vi "Disabled.vi"(7 "Robot Mode":T2, 10 "Match Info":T1={"Autonomous Elapsed Seconds"=0.0, "TeleOp Elapsed Seconds"=0.0, "Disabled Elapsed Seconds"=0.0, "Visited Autonomous"=FALSE, "Visited TeleOp"=FALSE, "Visited Disabled"=FALSE, "Autonomous Settings"={"Autonomous Style"=enum."Independent", "VI Refnum"=refnum}}, 11 "Call Context":T3) -> ()   [LabVIEW 2014]
doc: "This VI is called each time a disabled packet is received from the DS. It is often used to prepare for the next robot mode, to calibrate sensors, etc."
uses:
  <vilib>/Rock Robotics/WPI/DriverStation/WPI_DriverStationDerivedRobotMode.ctl
  <vilib>/Rock Robotics/WPI/DriverStation/WPI_DriverStationRobotMode2.ctl
  <vilib>/Rock Robotics/WPI/DriverStation/WPI_DriverStationMatch Info.ctl
  Raw Sequence Cluster.ctl
  LED Message.ctl
  LED_Patterns.ctl
  LED_Colors.ctl
  <vilib>/NI/AMC/Create Single Message.vi
  <vilib>/NI/AMC/Update Message Routing Info.vi
  <vilib>/NI/AMC/Send Message.vi
  <vilib>/Rock Robotics/WPI/Joystick/WPI_JoystickGetSetRefNum.vi
  <vilib>/NI/AMC/AMC.lvlib
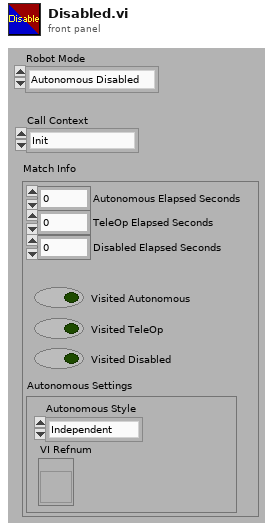
[diagram p1: front panel]
types:
  T1 = typedef "WPI_DriverStationMatch Info.ctl" = cluster{"Autonomous Elapsed Seconds":dbl, "TeleOp Elapsed Seconds":dbl, "Disabled Elapsed Seconds":dbl, "Visited Autonomous":bool, "Visited TeleOp":bool, "Visited Disabled":bool, "Autonomous Settings":cluster{"Autonomous Style":enum16{"Iterative", "Independent"}, "VI Refnum":refnum<vi>}}
  T2 = typedef "WPI_DriverStationRobotMode2.ctl" = enum16{"Autonomous Disabled", "Autonomous Enabled", "Teleop Disabled", "Teleop Enabled", "Disconnected", "Finish", "Test Disabled", "Test Enabled", "Emergency Stopped"}
  T3 = typedef "WPI_DriverStationDerivedRobotMode.ctl" = enum16{"Init", "Execute", "Stop"}
  T4 = typedef "Raw Sequence Cluster.ctl" = cluster{"Pattern":T5[], "Timing":u32[]}
  T5 = typedef "LED Message.ctl" = cluster{"Pattern":T6, "Color":T7, "Section":u8}
  T6 = typedef "LED_Patterns.ctl" = enum8{"Black White", "Solid", "Blink", "Sweep", "Sleep"}
  T7 = typedef "LED_Colors.ctl" = enum8{"Red", "Green", "Blue", "Cyan", "Magenta", "Yellow"}
  T8 = typedef "WPI_JoystickDevRef.ctl" = cluster{"Device":T9}
  T9 = typedef "WPI_JoystickDeviceEnum.ctl" = enum16{"USB 0", "USB 1", "USB 2", "USB 3", "USB 4", "USB 5"}
  T10 = typedef "AMC.lvlib/Message Queue.ctl" = refnum<queue>
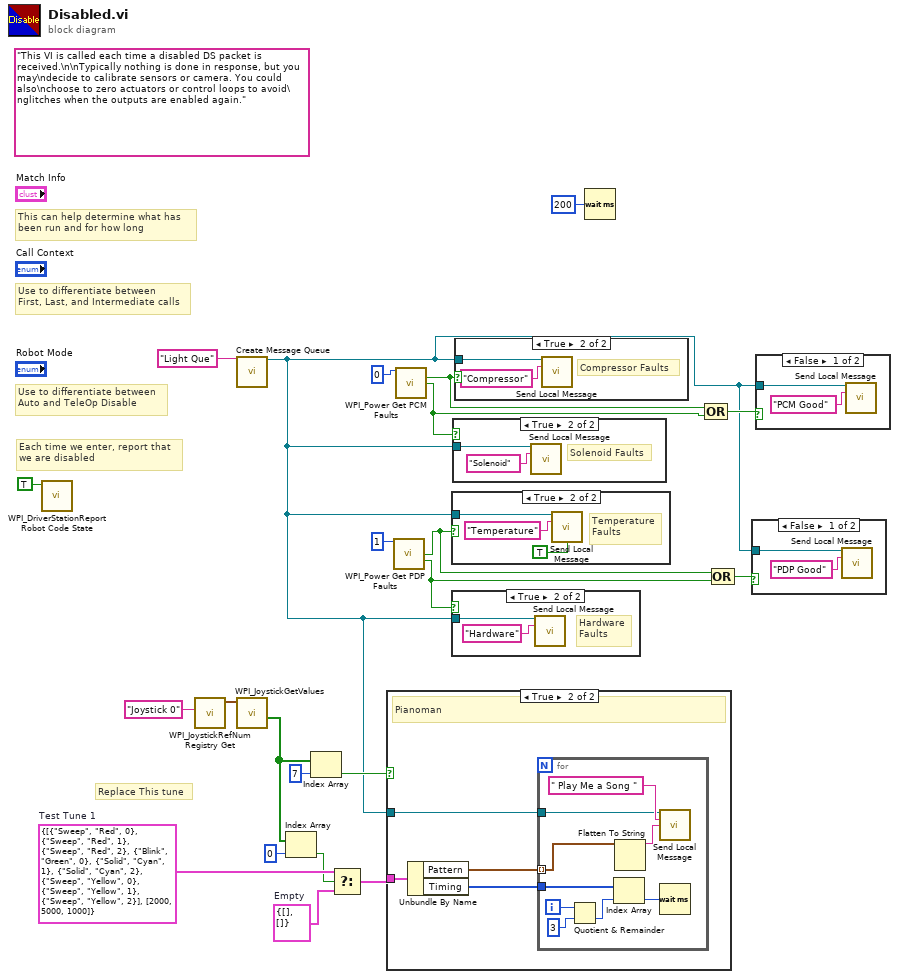
[diagram p0: block diagram]
diagram:
  w4 = T4 {"Pattern"=[], "Timing"=[]}  # Empty
  w6 = T4 {"Pattern"=[{"Pattern"=enum."Sweep", "Color"=enum."Red", "Section"=0}, {"Pattern"=enum."Sweep", "Color"=enum."Red", "Section"=1}, {"Pattern"=enum."Sweep", "Color"=enum."Red", "Section"=2}, {"Pattern"=enum."Blink", "Color"=enum."Green", "Section"=0}, {"Pattern"=enum."Solid", "Color"=enum."Cyan", "Section"=1}, {"Pattern"=enum."Solid", "Color"=enum."Cyan", "Section"=2}, {"Pattern"=enum."Sweep", "Color"=enum."Yellow", "Section"=0}, {"Pattern"=enum."Sweep", "Color"=enum."Yellow", "Section"=1}, {"Pattern"=enum."Sweep", "Color"=enum."Yellow", "Section"=2}], "Timing"=[2000, 5000, 1000]}  # Test Tune 1
  (unwired) "This VI is called each time a disabled DS packet is received.\n\nTypically nothing is done in response, but you may\ndecide to calibrate sensors or camera. You could also\nchoose to zero actuators or control loops to avoid\nglitches when the outputs are enabled again."
  # "Replace This tune"
  # "Each time we enter, report that\nwe are disabled"
  # "Use to differentiate between\nFirst, Last, and Intermediate calls"
  # "This can help determine what has\nbeen run and for how long"
  # "Use to differentiate between\nAuto and TeleOp Disable"
  n1 = call <vilib>:"WPI_DriverStationReport Robot Code State.vi"("Disabled"=TRUE ("Autonomous")) -> ()  [unwired: 10 in, 1 out]
  n2 = call <vilib>:"WPI_JoystickRefNum Registry Get.vi"("refnum name"="Joystick 0") -> ("JoystickDevRef"=w10:T8)  [unwired: 1 in, 9 out]
  n3 = call <vilib>:"Create Message Queue.vi"("message queue name"="Light Que") -> ("message queue out"=w7:T10)  [unwired: 13 in, 1 out]
  n4 = call <vilib>:"WPI_JoystickGetValues.vi"("JoystickDevRef"=w10) -> ("Buttons"=w1:bool[])  [unwired: 6 in, 4 out]
  n5 = Index Array(array=w1, index=0) -> (element=w2:bool)
  n6 = Index Array(array=w1, index=7) -> (element=w8:bool)
  n7 = Select(t=w6, s=w2, f=w4) -> (s? t:f=w5:T4)
  n8 = case shown="True" w8 {
    tunnel: w5 -> [_ w26]
    tunnel: w7 -> [_ w23]
    frame False {
    }
    frame True {
      # "Pianoman"
      n9 = Unbundle By Name(w26) -> ("Pattern"=w25:T5[], "Timing"=w24:u32[])
      n10 = for {
        tunnel: w25 -> [w28] mode=indexing
        tunnel: w24 -> [w33]
        tunnel: w23 -> [w29]
        i -> [w35]
        n11 = Quotient & Remainder(x=w35, y=3 ("Numeric")) -> (floor(x/y)=w32:i32)  [unwired: 1 out]
        n12 = Index Array(array=w33, index=w32) -> (element=w31:u32)
        n13 = Flatten To String(anything=w28) -> (data string=w27:string)  [unwired: 3 in, 2 out]
        n14 = call <vilib>:"Send Local Message.vi"("message queue in"=w29, "message name"=" Play Me a Song ", "message value"=w27) -> ()  [unwired: 10 in, 3 out]
        n15 = Wait (ms)(milliseconds to wait=w31) -> ()  [unwired: 1 out]
      }
    }
  }
  n16 = call <vilib>:"WPI_Power Get PDP Faults.vi"("Power Distribution Panel (0)"=u8 1) -> ("Temperature Fault"=w14:bool, "Hardware Fault"=w13:bool)  [unwired: 10 in, 3 out]
  n17 = call <vilib>:"WPI_Power Get PCM Faults.vi"("Pneumatics Control Module (0)"=u8 0) -> ("Compressor Fault"=w16:bool, "Solenoid Fault"=w18:bool)  [unwired: 11 in, 2 out]
  n18 = case shown="True" w14 {
    tunnel: w7 -> [_ w38]
    frame False {
    }
    frame True {
      # "Temperature\nFaults"
      n19 = call <vilib>:"Send Local Message.vi"("message queue in"=w38, "message name"="Temperature", "priority message (F)"=TRUE) -> ()  [unwired: 10 in, 3 out]
    }
  }
  n20 = case shown="True" w13 {
    tunnel: w7 -> [_ w40]
    frame False {
    }
    frame True {
      # "Hardware\nFaults"
      n21 = call <vilib>:"Send Local Message.vi"("message queue in"=w40, "message name"="Hardware") -> ()  [unwired: 11 in, 3 out]
    }
  }
  n22 = case shown="True" w18 {
    tunnel: w7 -> [_ w42]
    frame False {
    }
    frame True {
      # "Solenoid Faults"
      n23 = call <vilib>:"Send Local Message.vi"("message queue in"=w42, "message name"="Solenoid") -> ()  [unwired: 11 in, 3 out]
    }
  }
  n24 = case shown="True" w16 {
    tunnel: w7 -> [_ w44]
    frame False {
    }
    frame True {
      # "Compressor Faults"
      n25 = call <vilib>:"Send Local Message.vi"("message queue in"=w44, "message name"="Compressor") -> ()  [unwired: 11 in, 3 out]
    }
  }
  n26 = Wait (ms)(milliseconds to wait=u32 200) -> ()  [unwired: 1 out]
  n27 = Compound Arithmetic op=OR(w16, w18) -> (w17:bool)
  n28 = Compound Arithmetic op=OR(w14, w13) -> (w15:bool)
  n29 = case shown="False" w15 {
    tunnel: w7 -> [w45 _]
    frame False {
      n30 = call <vilib>:"Send Local Message.vi"("message queue in"=w45, "message name"="PDP Good") -> ()  [unwired: 11 in, 3 out]
    }
    frame True {
    }
  }
  n31 = case shown="False" w17 {
    tunnel: w7 -> [w47 _]
    frame False {
      n32 = call <vilib>:"Send Local Message.vi"("message queue in"=w47, "message name"="PCM Good") -> ()  [unwired: 11 in, 3 out]
    }
    frame True {
    }
  }
